vi "test_CCDAcquisitionSequenceImage.vi"(0 "device selection":enum16{"monochromator", "CCD", "SCD"}(ring)=enum."CCD", 1 "Test should pass":bool=TRUE, 5 "set-up a connection":bool=TRUE, 7 "set 3 ROIs / set 1 ROI":bool, 9 "tear down connection":bool=TRUE, 11 "error in":errorcluster, 12 "activate logger?":bool, 13 "Handler Name":string="example logger handler") -> (2 "ready":bool, 4 "results-JSON string":string, 6 "xyData":dbl[][][][](array[numeric]), 8 "meta data":T1[][](array[typedef]), 10 "log-file path":path, 15 "error out":errorcluster)   [LabVIEW 2023]
uses:
  <vilib>/addons/_JKI Toolkits/Caraya/classes/Test/Test.lvclass
  <vilib>/addons/_JKI Toolkits/Caraya/classes/Assert/Assert.lvclass
  Classes/CCD/CCD.lvclass
  Classes/CCD/XAxisConversionTypeEnum.ctl
  Classes/CCD/AcquisitionFormatEnum.ctl
  <vilib>/addons/_JKI Toolkits/Caraya/classes/Assert/Assert Not Error.vi
  Classes/CCD/CCDImageData.ctl
panel:
  # "Connector Pane"
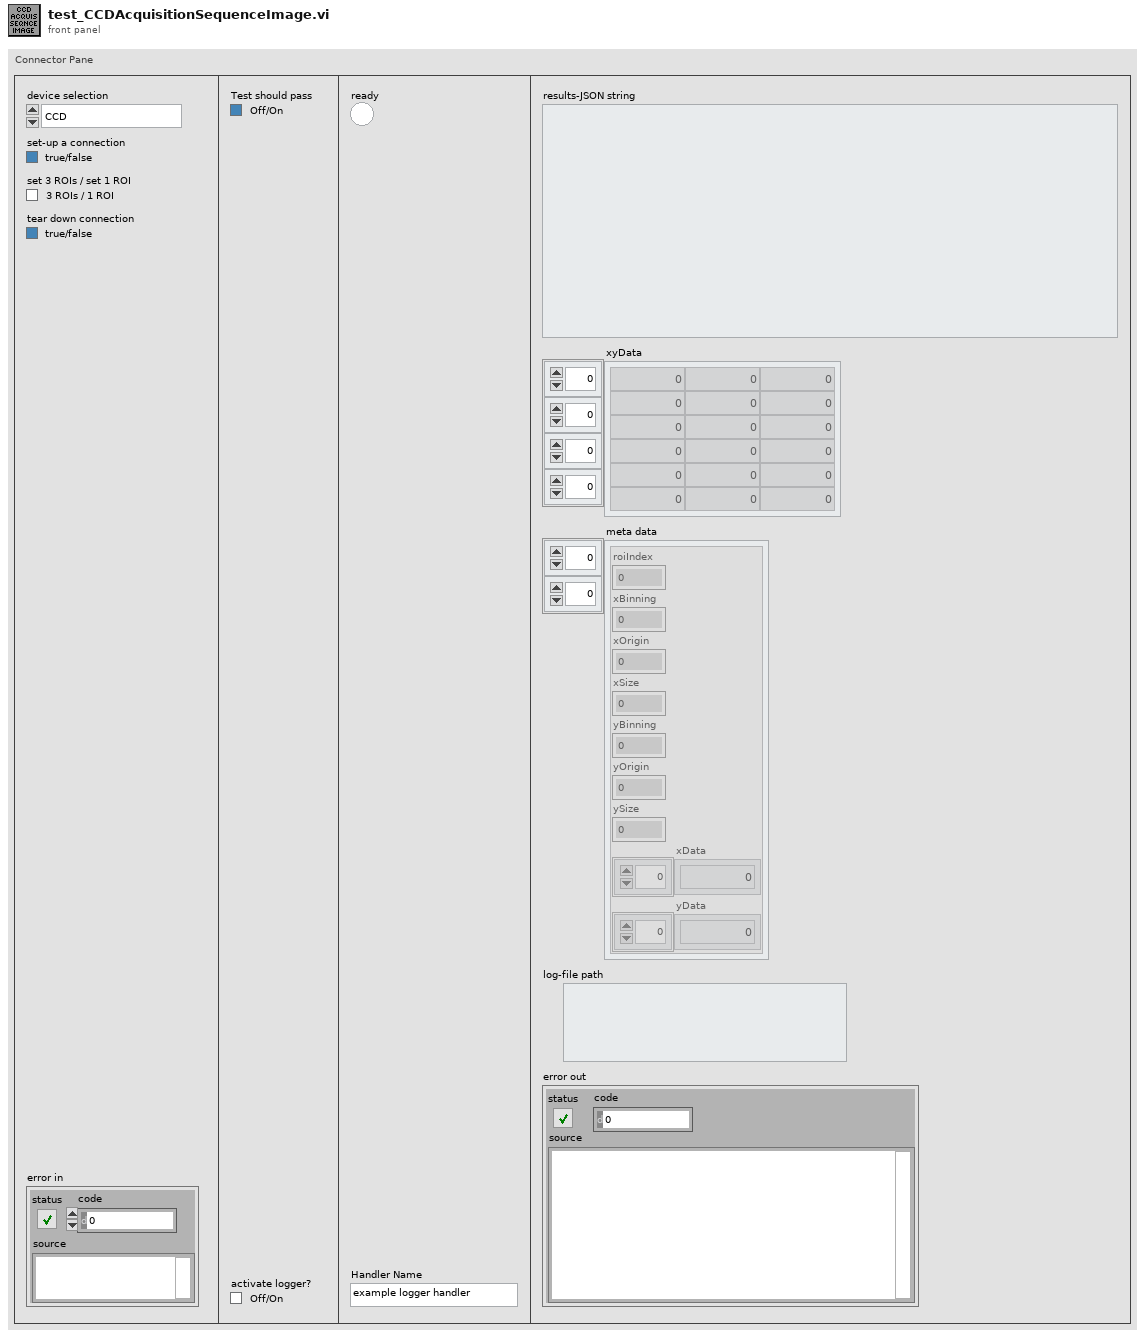
[diagram p1: front panel]
types:
  T1 = typedef "CCD.lvclass/CCDImageData.ctl" = cluster{"roiIndex":i32, "xBinning":i32, "xOrigin":i32, "xSize":i32, "yBinning":i32, "yOrigin":i32, "ySize":i32, "xData":dbl[], "yData":dbl[]}
  T2 = typedef "CCD.lvclass/AcquisitionFormatEnum.ctl" = enum16{"Spectra", "Image", "Crop", "Fast Kinetics"}
  T3 = typedef "CCD.lvclass/XAxisConversionTypeEnum.ctl" = enum16{"None (default)", "CCD FIT parameters contained in the CCD firmware", "Mono Wavelength parameters contained in the icl_settings.ini file"}
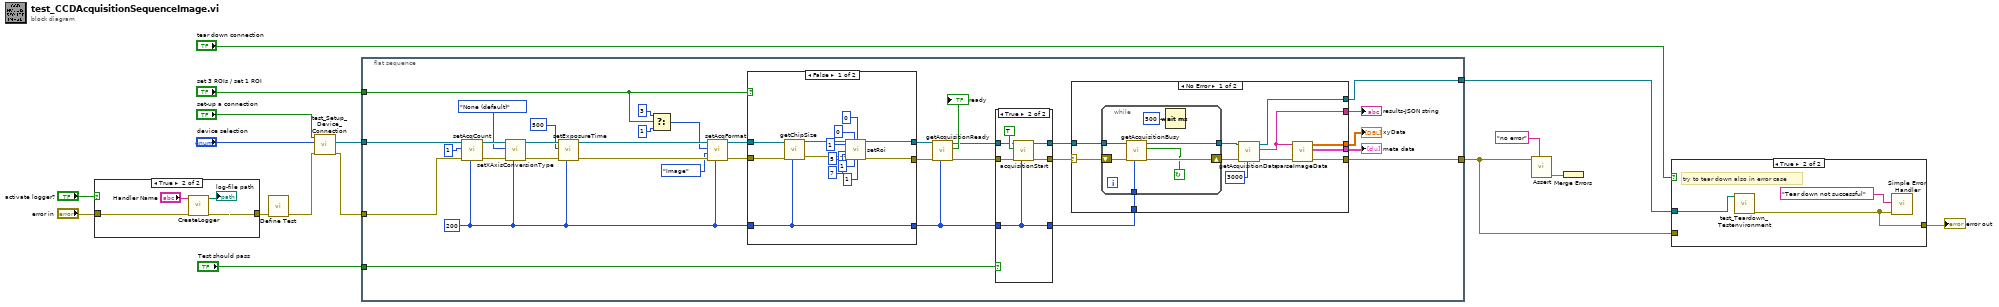
[diagram p0: block diagram]
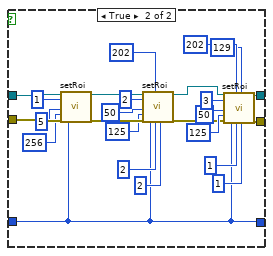
[diagram p2: hidden frame]
diagram:
  n1 = case shown="True" "activate logger?" {
    tunnel: [w17 w20] -> w2
    tunnel: "error in" -> [w17 w21]
    frame False {
    }
    frame True {
      n2 = call "CreateLogger.vi"("error in (no error)"=w21, "Handler Name"="Handler Name") -> ("error out"=w20:errorcluster, "log-file path"=→"log-file path":path)  [unwired: 8 in]
    }
  }
  n3 = call <vilib>:"Define Test.vi"("error in (no error)"=w2) -> ("error out"=w7:errorcluster)  [unwired: 9 in, 1 out]
  n4 = call "test_Setup_Device_Connection.vi"("error in (no error)"=w7, "device selection"="device selection", "set-up a connection"="set-up a connection") -> ("error out"=w8:errorcluster, "CCD.lvclass"=w9:refnum<class "CCD.lvclass">)  [unwired: 5 in, 2 out]
  n5 = flat-sequence {
    tunnel: w8 -> [w52]
    tunnel: w9 -> [w53]
    tunnel: [w40] -> w12
    tunnel: "Test should pass" -> [w54]
    tunnel: [w41] -> w11
    tunnel: "set 3 ROIs / set 1 ROI" -> [w33]
    frame #0 {
      w25 = 200 ("Delay between send and receive [ms]")
      n6 = call "setAcqCount.vi"("Delay between send and receive [ms]"=w25, "error in (no error)"=w52, "count"=1, "CCD in"=w53) -> ("error out"=w49:errorcluster, "CCD out"=w50:refnum<class "CCD.lvclass">)  [unwired: 4 in, 2 out]
      n7 = call "setXAxisConversionType.vi"("Delay between send and receive [ms]"=w25, "error in (no error)"=w49, "type"=XAxisConversionTypeEnum."None (default)" ("Enum"), "CCD in"=w50) -> ("error out"=w47:errorcluster, "CCD out"=w46:refnum<class "CCD.lvclass">)  [unwired: 4 in, 2 out]
      n8 = call "setExposureTime.vi"("Delay between send and receive [ms]"=w25, "error in (no error)"=w47, "exposure time [ms] or [us]"=500 ("exposure time [ms]"), "CCD in"=w46) -> ("error out"=w43:errorcluster, "CCD out"=w44:refnum<class "CCD.lvclass">)  [unwired: 4 in, 2 out]
      n9 = Select(t=3 ("number of ROIs"), s=w33, f=1) -> (s? t:f=w30:i32)
      n10 = call "setAcqFormat.vi"("Delay between send and receive [ms]"=w25, "error in (no error)"=w43, "format"=AcquisitionFormatEnum."Image" ("acquisition format"), "number of ROIs"=w30, "CCD in"=w44) -> ("error out"=w36:errorcluster, "CCD out"=w37:refnum<class "CCD.lvclass">)  [unwired: 3 in, 2 out]
      n11 = case shown="False" w33 {
        tunnel: w37 -> [w66 w93]
        tunnel: w36 -> [w67 w92]
        tunnel: w25 -> [w68 w71]
        tunnel: [w68 w71] -> _
        tunnel: [w60 w70] -> w35
        tunnel: [w61 w69] -> w34
        frame False {
          n12 = call-dynamic "getChipSize.vi"("Delay between send and receive [ms]"=w68, "error in (no error)"=w67, "CCD in"=w66) -> ("error out"=w62:errorcluster, "CCD out"=w59:refnum<class "CCD.lvclass">)  [unwired: 5 in, 2 out]
          n13 = call "setRoi.vi"("CCD in"=w59, "ROI-index"=1, "xSize"=5, "ySize"=7, "error in (no error)"=w62, "xOrigin"=0, "xBin"=1, "yOrigin"=0, "yBin"=1) -> ("CCD out"=w60:refnum<class "CCD.lvclass">, "error out"=w61:errorcluster)  [unwired: 7 in, 2 out]
        }
        frame True {
          n14 = call "setRoi.vi"("CCD in"=w93, "ROI-index"=1, "xSize"=5, "ySize"=256, "error in (no error)"=w92, "Delay between send and receive [ms]"=w71) -> ("CCD out"=w91:refnum<class "CCD.lvclass">, "error out"=w90:errorcluster)  [unwired: 10 in, 2 out]
          n15 = call "setRoi.vi"("CCD in"=w91, "ROI-index"=2, "xSize"=50, "ySize"=125, "error in (no error)"=w90, "Delay between send and receive [ms]"=w71, "xOrigin"=202, "xBin"=2, "yBin"=2) -> ("CCD out"=w76:refnum<class "CCD.lvclass">, "error out"=w75:errorcluster)  [unwired: 7 in, 2 out]
          n16 = call "setRoi.vi"("CCD in"=w76, "ROI-index"=3, "xSize"=50, "ySize"=125, "error in (no error)"=w75, "Delay between send and receive [ms]"=w71, "xOrigin"=202, "xBin"=1, "yOrigin"=129, "yBin"=1) -> ("CCD out"=w70:refnum<class "CCD.lvclass">, "error out"=w69:errorcluster)  [unwired: 6 in, 2 out]
        }
      }
      n17 = call "getAcquisitionReady.vi"("Delay between send and receive [ms]"=w25, "error in (no error)"=w34, "CCD in"=w35) -> ("error out"=w29:errorcluster, "ready"=→"ready":bool, "CCD out"=w26:refnum<class "CCD.lvclass">)  [unwired: 6 in]
      n18 = case shown="True" w54 {
        tunnel: w26 -> [w116 w122]
        tunnel: w29 -> [w117 w121]
        tunnel: [w116 w119] -> w28
        tunnel: [w117 w120] -> w27
        tunnel: w25 -> [w115 w118]
        tunnel: [w115 w118] -> w22
        frame False {
        }
        frame True {
          n19 = call "acquisitionStart.vi"("Delay between send and receive [ms]"=w118, "error in (no error)"=w121, "openShutter"=TRUE, "CCD in"=w122) -> ("error out"=w120:errorcluster, "CCD out"=w119:refnum<class "CCD.lvclass">)  [unwired: 4 in, 2 out]
        }
      }
      n20 = case shown="No Error" w27 {
        selector: w27 -> [w102 w113]
        tunnel: w28 -> [w105 w114]
        tunnel: [w101 w114] -> w41
        tunnel: [w99 w113] -> w40
        tunnel: [w98 _] -> w39
        tunnel: [w96 _] -> w24
        tunnel: [w97 _] -> w23
        tunnel: w22 -> [w94 _]
        frame No Error {
          n21 = while {
            tunnel: w105 -> [w112]
            tunnel: [w111] -> w104
            shift-right: [w109] -> w103
            shift-left: w102 -> [w108]
            tunnel: w94 -> [w106]
            stop <- w107 continue-if-true
            n22 = call "getAcquisitionBusy.vi"("Delay between send and receive [ms]"=w106, "error in (no error)"=w108, "CCD in"=w112) -> ("error out"=w109:errorcluster, "isBusy"=w107:bool, "CCD out"=w111:refnum<class "CCD.lvclass">)  [unwired: 6 in]
            n23 = Wait (ms)(milliseconds to wait=u32 500) -> ()  [unwired: 1 out]
          }
          n24 = call "getAcquisitionData.vi"("Delay between send and receive [ms]"=3000, "error in (no error)"=w103, "CCD in"=w104) -> ("error out"=w100:errorcluster, "results-JSON string"=w98:string, "CCD out"=w101:refnum<class "CCD.lvclass">)  [unwired: 6 in]
          n25 = call "parseImageData.vi"("error in (no error)"=w100, "results-JSON string"=w98) -> ("error out"=w99:errorcluster, "meta data"=w97:T1[][], "xyData"=w96:dbl[][][][])  [unwired: 7 in]
        }
        frame Error {
        }
      }
      "results-JSON string" <- w39
      "xyData" <- w24
      "meta data" <- w23
    }
  }
  n26 = call-poly <vilib>:"Assert.vi"("Label"="no error" ("Label (VI Title)"), "Not Error?"=w12) -> ("error out"=w14:errorcluster)  [unwired: 8 in, 1 out]
  n27 = Merge Errors(w14) -> ()  [unwired: 1 out]
  n28 = case shown="True" "tear down connection" {
    tunnel: w11 -> [_ w126]
    tunnel: [w124 w125] -> w10
    tunnel: w12 -> [w124 _]
    frame False {
    }
    frame True {
      # "try to tear down also in error case"
      n29 = call "test_Teardown_Testenvironment.vi"("GenericDevice.lvclass"=w126) -> ("error out"=w125:errorcluster)  [unwired: 9 in, 1 out]
      n30 = call <vilib>:"Simple Error Handler.vi"("error source (\" \")"="Tear down not successful" ("error source (\" \")"), "error in (no error)"=w125) -> ()  [unwired: 3 in, 5 out]
    }
  }
  "error out" <- w10
